vi "DIC main 11082010.vi"() -> ()   [LabVIEW 2010]
panel:
  in  "File Header Settings":T1={"Flow Rate"="", "Sample Volume"="", "Operator"="", "Sample Type"="Unknown"}
  in  "Sample Port":u16(ring) items=["A"=1, "B"=2, "C"=3, "D"=4, "E"=5, "F"=6, "G"=7, "H"=8]
  in  "flush syringe":bool
  in  "flush acid":bool
  in  "Syringe Flushes":i32=3
  out "file error out":errorcluster
  out "LiCor errors out":errorcluster
  out "kloehn errors out":errorcluster
  out "relay errors out":errorcluster
  out "Final Integral":dbl
  out "CO2 Integral":dbl
  out "pCO2_start":dbl
  out "pCO2_end":dbl
  in  "Start Run":bool caption="Make all inputs are set before hitting start!!!"
  in  "Number of Repeats":i32=1
  in  "stop":bool
  out "pCO2":dbl
  in  "Data Directory":path
  # "DIC Analysis Tool"
  # "Locate the directory where you would like to place your data files and then click \"Current Folder\""
  # "Global variables in Gernot's code:\nCO2pres\nCO2_Temp\nCom_Error\nCurrentRepeat\nDataFile\nError_Log\nH2O\nLicorData\nOperation\npCO2\npCO2_end\npCO2_integrate\npCO2_max\npCO2_start\nPeakAvg\nPeakRead\nRepeat\nSampleCount\nSampleID\nSampleTime\nSampleType\nSequenceTime\nSyringeCom\nTCO2Error\nValvePosition\nXplot\nYplot"
  # "Number of flushes before a sample is run or when Flush Syringe is pressed."
  # "Critical Points"
  # "Real Time"
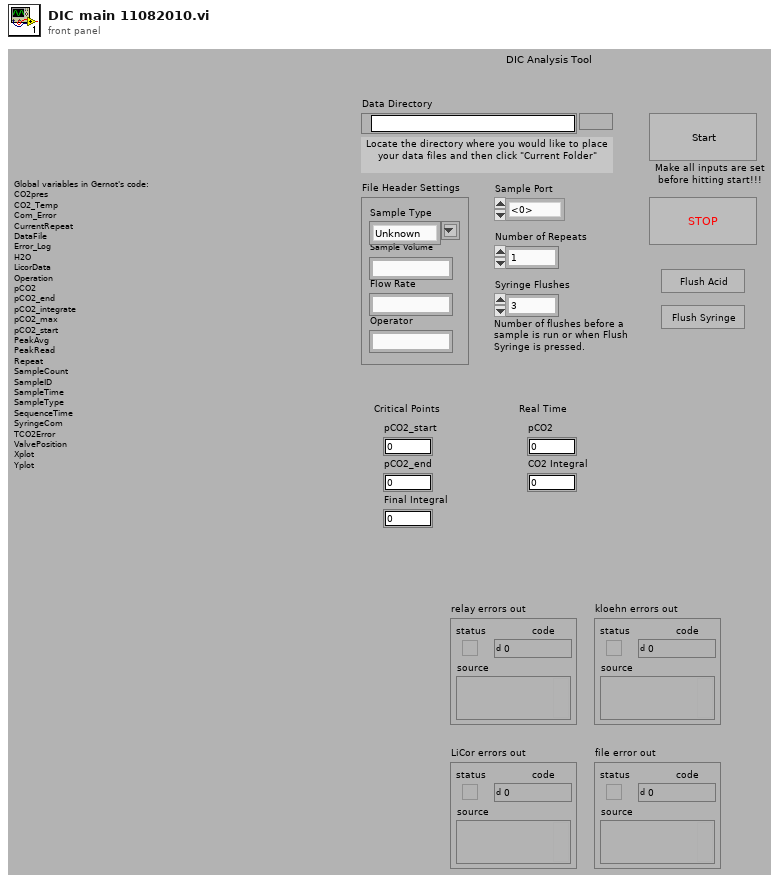
[diagram p1: front panel]
types:
  T1 = cluster{"Flow Rate":string, "Sample Volume":string, "Operator":string, "Sample Type":string}
  T2 = cluster{"baud rate (9600)":u32, "data bits (8)":u16, "parity (0:none)":enum16{"None", "Odd", "Even", "Mark", "Space"}, "stop bits (10: 1 bit)":u16, "flow control (0:none)":u16, "timeout (10sec)":u32, "termination char\n(0xA = '\\n' = LF) ":u8, "Enable Termination\nChar (T)":bool}
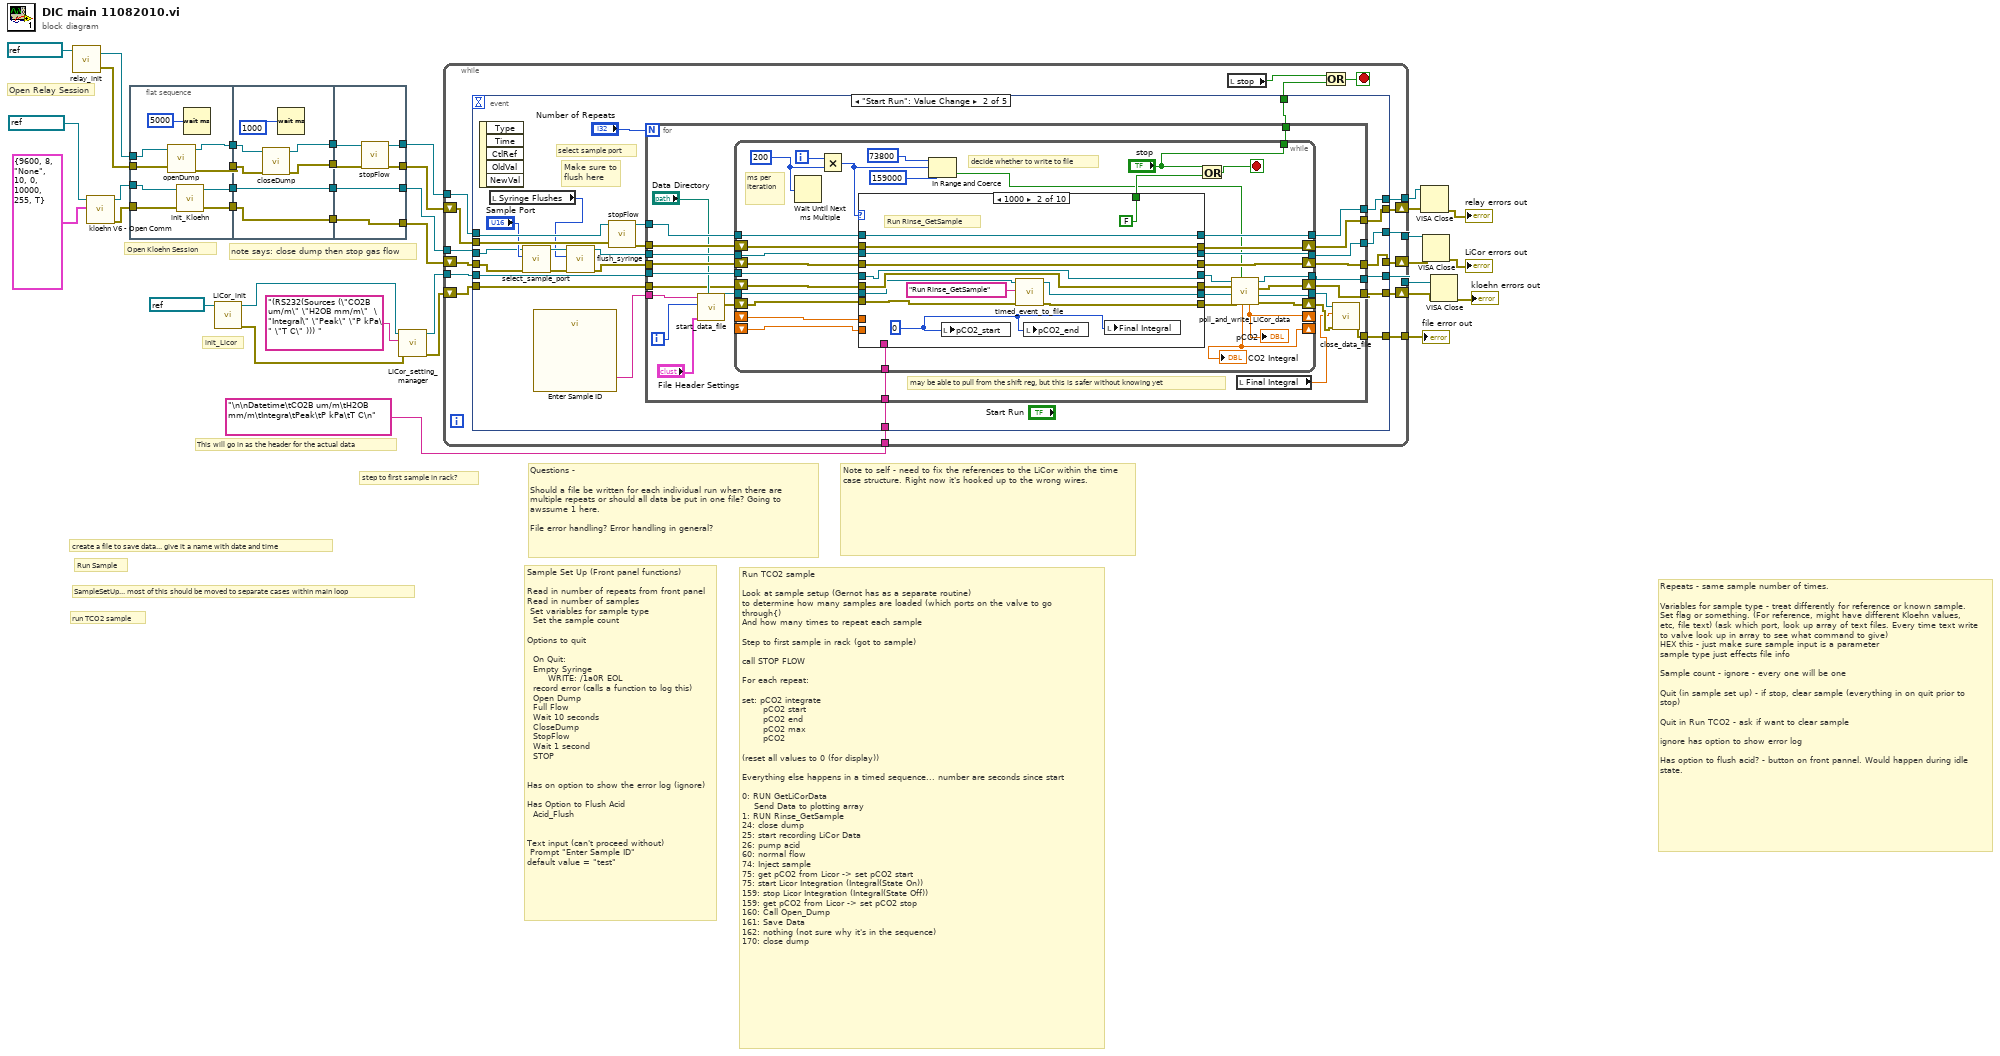
[diagram p0: block diagram]
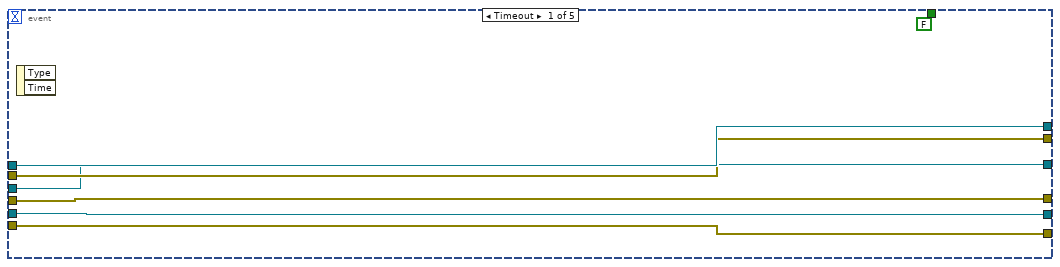
[diagram p2: hidden frame]
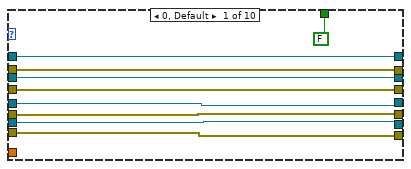
[diagram p3: hidden frame]
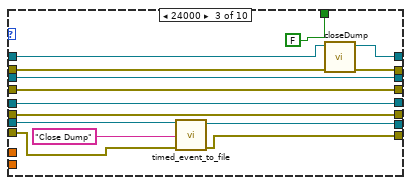
[diagram p4: hidden frame]
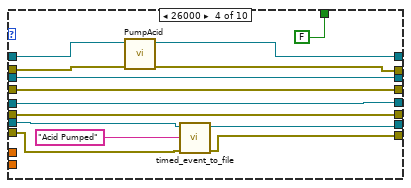
[diagram p5: hidden frame]
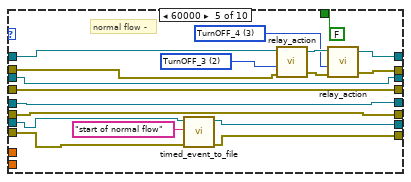
[diagram p6: hidden frame]
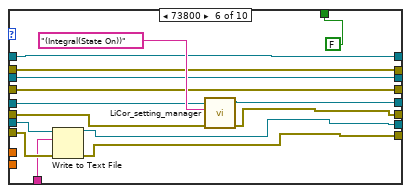
[diagram p7: hidden frame]
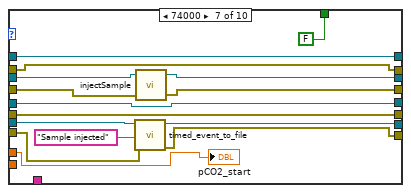
[diagram p8: hidden frame]
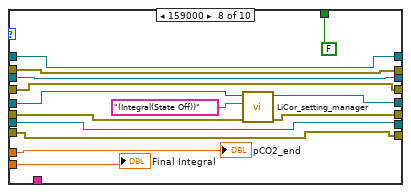
[diagram p9: hidden frame]
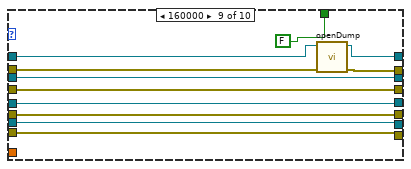
[diagram p10: hidden frame]
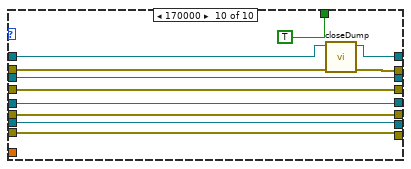
[diagram p11: hidden frame]
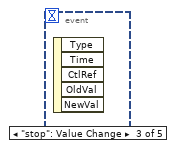
[diagram p12: hidden frame]
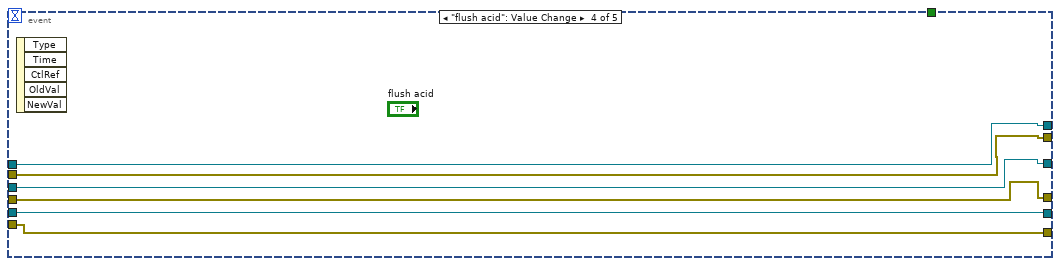
[diagram p13: hidden frame]
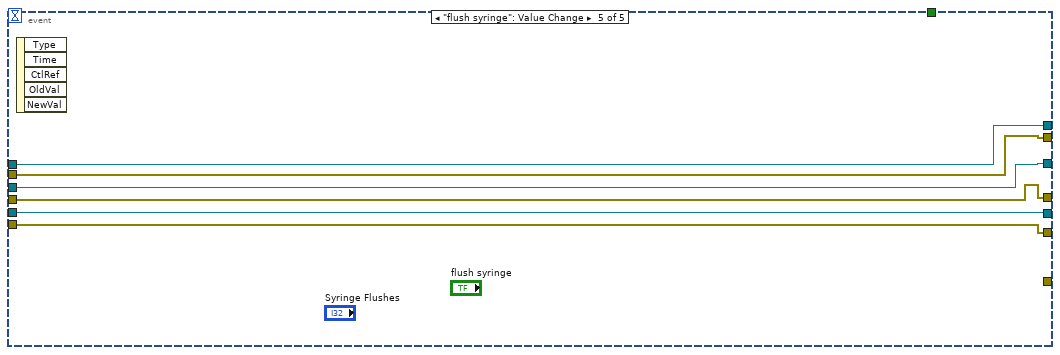
[diagram p14: hidden frame]
diagram:
  # "This will go in as the header for the actual data"
  # "step to first sample in rack?"
  # "Note to self - need to fix the references to the LiCor within the time case structure. Right now it's hooked up to the wrong wires."
  # "Questions - \n\nShould a file be written for each individual run when there are multiple repeats or should all data be put in one file? Going to awssume 1 here.\n\nFile error handling? Error handling in general?"
  # "Repeats - same sample number of times.\n\nVariables for sample type - treat differently for reference or known sample. Set flag or something. (For reference, might have different Kloehn values, etc, file text) (ask which port, look up array of text files. Every time text write to valve look up in array to see what command to give) \nHEX this - just make sure sample input is a parameter\nsample type just effects file info\n\nSample count - ignore - every one will be one\n\nQuit (in sample set up) - if stop, clear sample (everything in on quit prior to stop)\n\nQuit in Run TCO2 - ask if want to clear sample\n\nignore has option to show error log\n\nHas option to flush acid? - button on front pannel. Would happen during idle state."
  # "create a file to save data... give it a name with date and time"
  # "init_Licor"
  # "Run Sample"
  # "run TCO2 sample"
  # "SampleSetUp... most of this should be moved to separate cases within main loop"
  # "note says: close dump then stop gas flow"
  # "Open Relay Session"
  # "Open Kloehn Session"
  # "Run TCO2 sample\n\nLook at sample setup (Gernot has as a separate routine)\nto determine how many samples are loaded (which ports on the valve to go through{)\nAnd how many times to repeat each sample\n\nStep to first sample in rack (got to sample)\n\ncall STOP FLOW\n\nFor each repeat:\n\nset: pCO2 integrate\n       pCO2 start\n       pCO2 end\n       pCO2 max\n       pCO2 \n\n(reset all values to 0 (for display))\n\nEverything else happens in a timed sequence... number are seconds since start\n\n0: RUN GetLiCorData\n    Send Data to plotting array\n1: RUN Rinse_GetSample\n24: close dump\n25: start recording LiCor Data\n26: pump acid\n60: normal flow\n74: Inject sample\n75: get pCO2 from Licor -> set pCO2 start\n75: start Licor Integration (Integral(State On))\n159: stop Licor Integration (Integral(State Off))\n159: get pCO2 from Licor -> set pCO2 stop\n160: Call Open_Dump\n161: Save Data\n162: nothing (not sure why it's in the sequence)\n170: close dump"
  # "Sample Set Up (Front panel functions)\n\nRead in number of repeats from front panel\nRead in number of samples \n Set variables for sample type\n  Set the sample count\n\nOptions to quit\n\n  On Quit:\n  Empty Syringe \n       WRITE: /1a0R EOL\n  record error (calls a function to log this)\n  Open Dump\n  Full Flow\n  Wait 10 seconds\n  CloseDump\n  StopFlow\n  Wait 1 second\n  STOP\n\n\nHas on option to show the error log (ignore)\n\nHas Option to Flush Acid\n  Acid_Flush\n\n\nText input (can't proceed without)\n Prompt \"Enter Sample ID\"\ndefault value = \"test\""
  n1 = call "relay_init.vi"("VISA resource in"=refnum<visa-resource-name> "COM12" ("Koehn VISA Ref")) -> ("error out"=w35:errorcluster, "VISA resource out"=w36:refnum<visa-resource-name>)  [unwired: 2 in]
  n2 = call "kloehn V6 - Open Comm .vi"("Serial Parameters"=T2 {"baud rate (9600)"=9600, "data bits (8)"=8, "parity (0:none)"=enum."None", "stop bits (10: 1 bit)"=10, "flow control (0:none)"=0, "timeout (10sec)"=10000, "termination char\n(0xA = '\\n' = LF) "=255, "Enable Termination\nChar (T)"=TRUE} ("Port Configuration"), "VISA Ref in"=refnum<visa-resource-name> "COM10" ("Koehn VISA Ref")) -> ("error out"=w30:errorcluster, "VISA Ref out"=w31:refnum<visa-resource-name>)  [unwired: 8 in]
  n3 = flat-sequence {
    tunnel: w36 -> [w45]
    tunnel: w35 -> [w44]
    tunnel: [w43] -> w34
    tunnel: [w42] -> w33
    tunnel: w31 -> [w41]
    tunnel: w30 -> [w40]
    tunnel: [w39] -> w29
    tunnel: [w38] -> w28
    tunnel: w34 -> [w52]
    tunnel: w33 -> [w51]
    tunnel: w29 -> [w47]
    tunnel: w28 -> [w46]
    tunnel: [w50] -> w25
    tunnel: [w49] -> w24
    tunnel: [w47] -> w15
    tunnel: [w46] -> w14
    tunnel: w25 -> [w57]
    tunnel: w24 -> [w58]
    tunnel: [w56] -> w17
    tunnel: [w55] -> w16
    tunnel: w15 -> [w54]
    tunnel: w14 -> [w53]
    tunnel: [w54] -> w13
    tunnel: [w53] -> w12
    frame #0 {
      n4 = call "openDump.vi"("error in"=w44, "VISA resource name"=w45) -> ("error out"=w42:errorcluster, "VISA resource out"=w43:refnum<visa-resource-name>)  [unwired: 8 in]
      n5 = call "init_Kloehn.vi"("error in"=w40, "VISA resource in"=w41) -> ("error out"=w38:errorcluster, "VISA resource out"=w39:refnum<visa-resource-name>)  [unwired: 2 in]
      n6 = Wait (ms)(milliseconds to wait=5000) -> ()  [unwired: 1 out]
    }
    frame #1 {
      n7 = call "closeDump.vi"("error in"=w51, "VISA resource name"=w52) -> ("error out"=w50:errorcluster, "VISA resource out"=w49:refnum<visa-resource-name>)  [unwired: 8 in]
      n8 = Wait (ms)(milliseconds to wait=1000) -> ()  [unwired: 1 out]
    }
    frame #2 {
      n9 = call "stopFlow.vi"("error in"=w57, "VISA resource name"=w58) -> ("error out"=w55:errorcluster, "VISA resource out"=w56:refnum<visa-resource-name>)  [unwired: 8 in]
    }
  }
  n10 = call "LiCor_init.vi"("VISA resource name"=refnum<visa-resource-name> "COM11" ("Koehn VISA Ref")) -> ("error out"=w20:errorcluster, "VISA out"=w21:refnum<visa-resource-name>)  [unwired: 9 in]
  n11 = call "LiCor_setting_manager.vi"("error in"=w20, "string to write"="(RS232(Sources (\"CO2B um/m\" \"H2OB mm/m\"  \"Integral\" \"Peak\" \"P kPa\" \"T C\" ))) " ("String"), "VISA session in"=w21) -> ("error out"=w18:errorcluster, "VISA session out"=w19:refnum<visa-resource-name>)  [unwired: 7 in]
  n12 = while {
    tunnel: w19 -> [w63]
    tunnel: w17 -> [w75]
    tunnel: w13 -> [w73]
    tunnel: [w69] -> w10
    tunnel: [w68] -> w9
    tunnel: [w66] -> w7
    tunnel: "\n\nDatetime\tCO2B um/m\tH2OB mm/m\tIntegra\tPeak\tP kPa\tT C\n" -> [w60]
    tunnel: [w59] -> w4
    shift-right: [w70] -> w11
    shift-left: w18 -> [w64]
    shift-right: [w65] -> w6
    shift-left: w12 -> [w72]
    shift-right: [w67] -> w8
    shift-left: w16 -> [w74]
    stop <- w71 stop-if-true
    n13 = event shown="[1] \"Start Run\": Value Change" {
      selector: _ -> [_ _ _ _ _]
      dyn-events: _ -> [_ _ _ _ _]
      timeout: _ -> [_ _ _ _ _]
      tunnel: w63 -> [w81 w106 _ w301 w307]
      tunnel: w64 -> [w82 w105 _ w300 w306]
      tunnel: w75 -> [w80 w102 _ w305 w311]
      tunnel: w74 -> [w79 w101 _ w304 w310]
      tunnel: w73 -> [w78 w89 _ w303 w309]
      tunnel: w72 -> [w77 w88 _ w302 w308]
      tunnel: [FALSE w100 _ _ _] -> w61
      tunnel: [w82 w99 _ w300 w306] -> w70
      tunnel: [w81 w94 _ w301 w307] -> w69
      tunnel: [w80 w98 _ w305 w311] -> w68
      tunnel: [w79 w97 _ w304 w310] -> w67
      tunnel: [w78 w96 _ w303 w309] -> w66
      tunnel: [w77 w95 _ w302 w308] -> w65
      tunnel: w60 -> [_ w93 _ _ _]
      tunnel: [_ w91 _ _ _] -> w59
      event Timeout {
        n14 = event-data() -> ()  [unwired: 1 in, 2 out]
      }
      event "Start Run": Value Change {
        # "select sample port"
        # "Make sure to flush here"
        n15 = event-data() -> ()  [unwired: 1 in, 5 out]
        n16 = local read "Syringe Flushes"() -> (w83:i32)
        n17 = call "select_sample_port.vi"("error in"=w88, "Sample Port"="Sample Port", "VISA resource in"=w89) -> ("error out"=w87:errorcluster, "VISA resource out"=w86:refnum<visa-resource-name>)  [unwired: 7 in]
        n18 = call "Enter Sample ID"() -> ("sample id"=w92:string)  [unwired: 17 in, 2 out]
        n19 = call "flush_syringe.vi"("error in"=w87, "Syringe Flushes"=w83, "VISA resource in"=w86) -> ("error out"=w84:errorcluster, "VISA resource out"=w85:refnum<visa-resource-name>)  [unwired: 7 in]
        n20 = call "stopFlow.vi"("error in"=w101, "VISA resource name"=w102) -> ("error out"=w103:errorcluster, "VISA resource out"=w104:refnum<visa-resource-name>)  [unwired: 8 in]
        n21 = for {
          N: "Number of Repeats" -> [_]
          tunnel: w106 -> [w131]
          tunnel: w105 -> [w113]
          tunnel: w104 -> [w129]
          tunnel: w103 -> [w130]
          tunnel: [w128] -> w100
          tunnel: w85 -> [w127]
          tunnel: w84 -> [w126]
          tunnel: [w125] -> w99
          tunnel: [w124] -> w98
          tunnel: [w123] -> w97
          tunnel: [w122] -> w96
          tunnel: [w121] -> w95
          tunnel: [w120] -> w94
          tunnel: w92 -> [w116]
          tunnel: w93 -> [w117]
          tunnel: [w109] -> w91
          i -> [w114]
          # "may be able to pull from the shift reg, but this is safer without knowing yet"
          n22 = call "start_data_file.vi"("DataFile"="Data Directory", "File Header Settings"="File Header Settings", "iteration"=w114, "sample id"=w116) -> ("error out"=w118:errorcluster, "Byte Stream File Refnum"=w119:refnum<file>)  [unwired: 6 in]
          n23 = while {
            tunnel: w131 -> [w151]
            shift-right: [w140] -> w125
            shift-left: w113 -> [w150]
            tunnel: w129 -> [w165]
            shift-right: [w138] -> w111
            shift-left: w118 -> [w148]
            tunnel: ["stop"] -> w128
            tunnel: w127 -> [w163]
            shift-right: [w161] -> w121
            shift-left: w126 -> [w162]
            tunnel: [w160] -> w122
            tunnel: [w159] -> w124
            shift-right: [w158] -> w123
            shift-left: w130 -> [w164]
            tunnel: [w141] -> w120
            tunnel: w119 -> [w149]
            tunnel: [w139] -> w112
            tunnel: w117 -> [w152]
            shift-right: [w135] -> _
            shift-left: _ -> [w134]
            shift-right: [w133] -> _
            shift-left: _ -> [w132]
            i -> [w157]
            stop <- w153 stop-if-true
            w156 = 200 ("ms between samples")
            # "decide whether to write to file"
            # "ms per iteration"
            n24 = Wait Until Next ms Multiple(millisecond multiple=w156) -> ()  [unwired: 1 out]
            n25 = Multiply(x=w157, y=w156) -> (x*y=w136:i32)
            n26 = case shown="1000" w136 {
              tunnel: w165 -> [w166 w185 w199 w213 w225 w239 w263 w274 w286 w297]
              tunnel: w164 -> [w172 w184 w197 w212 w224 w240 w262 w273 w285 w296]
              tunnel: w163 -> [w174 w187 w200 w215 w233 w241 w261 w277 w288 w299]
              tunnel: w162 -> [w173 w186 w201 w214 w232 w242 w260 w276 w287 w298]
              tunnel: [w173 w186 w201 w214 w232 w242 w258 w276 w287 w298] -> w161
              tunnel: [w174 w187 w200 w215 w233 w241 w259 w277 w288 w299] -> w160
              tunnel: [w166 w185 w198 w211 w223 w239 w263 w274 w283 w294] -> w159
              tunnel: [w172 w184 w196 w210 w222 w240 w262 w273 w284 w295] -> w158
              tunnel: w151 -> [w170 w183 w195 w209 w231 w244 w256 w272 w282 w293]
              tunnel: w150 -> [w169 w182 w194 w208 w230 w243 w257 w271 w281 w292]
              tunnel: [w169 w182 w194 w208 w230 w236 w257 w269 w281 w292] -> w142
              tunnel: [w170 w183 w195 w209 w231 w237 w256 w270 w282 w293] -> w144
              tunnel: w149 -> [w168 w180 w191 w205 w219 w246 w253 w267 w279 w290]
              tunnel: [w167 w178 w188 w202 w217 w234 w250 w266 w278 w289] -> w143
              tunnel: w148 -> [w167 w179 w190 w204 w216 w248 w252 w266 w278 w289]
              tunnel: [w168 w177 w189 w203 w218 w235 w251 w267 w279 w290] -> w145
              tunnel: [FALSE FALSE FALSE FALSE FALSE FALSE FALSE FALSE FALSE TRUE] -> w155
              tunnel: w152 -> [_ _ _ _ _ w247 _ _ _ _]
              tunnel: w134 -> [_ _ _ _ _ _ w249 w265 _ _]
              tunnel: w132 -> [_ _ _ _ _ _ _ w264 _ _]
              frame 0, Default {
              }
              frame 1000 {
                w175 = 0
                # "Run Rinse_GetSample"
                n27 = local write "pCO2_start"(w175) -> ()
                n28 = call "timed_event_to_file.vi"("file error in"=w179, "String"="Run Rinse_GetSample", "file ref in"=w180) -> ("file error out"=w178:errorcluster, "file ref out"=w177:refnum<file>)  [unwired: 7 in]
                n29 = local write "pCO2_end"(w175) -> ()
                n30 = local write "Final Integral"(w175) -> ()
              }
              frame 24000 {
                n31 = call "timed_event_to_file.vi"("file error in"=w190, "String"="Close Dump", "file ref in"=w191) -> ("file error out"=w188:errorcluster, "file ref out"=w189:refnum<file>)  [unwired: 7 in]
                n32 = call "closeDump.vi"("error in"=w197, "VISA resource name"=w199) -> ("error out"=w196:errorcluster, "VISA resource out"=w198:refnum<visa-resource-name>)  [unwired: 8 in]
              }
              frame 26000 {
                n33 = call "PumpAcid.vi"("error in"=w212, "VISA resource name"=w213) -> ("error out"=w210:errorcluster, "VISA resource out"=w211:refnum<visa-resource-name>)  [unwired: 8 in]
                n34 = call "timed_event_to_file.vi"("file error in"=w204, "String"="Acid Pumped", "file ref in"=w205) -> ("file error out"=w202:errorcluster, "file ref out"=w203:refnum<file>)  [unwired: 7 in]
              }
              frame 60000 {
                w226 = u8 3 items=["TurnON_1"=8, "TurnON_PUMP"=9, "TurnON_3"=10, "TurnON_4"=11, "CLOSE DUMP OFF_1"=0, "TurnOFF_PUMP"=1, "TurnOFF_3"=2, "TurnOFF_4"=3, "OpenAll"=30, "CloseAllRelay"=29] ("Action 2")
                w229 = u8 2 items=["TurnON_1"=8, "TurnON_PUMP"=9, "TurnON_3"=10, "TurnON_4"=11, "CLOSE DUMP OFF_1"=0, "TurnOFF_PUMP"=1, "TurnOFF_3"=2, "TurnOFF_4"=3, "OpenAll"=30, "CloseAllRelay"=29] ("Action")
                # "normal flow -"
                n35 = call "timed_event_to_file.vi"("file error in"=w216, "String"="start of normal flow", "file ref in"=w219) -> ("file error out"=w217:errorcluster, "file ref out"=w218:refnum<file>)  [unwired: 7 in]
                n36 = call "relay_action.vi"("VISA resource in"=w225, "Action"=w229, "error in"=w224) -> ("VISA resource out"=w228:refnum<visa-resource-name>, "error out"=w227:errorcluster)  [unwired: 4 in]
                n37 = call "relay_action.vi"("VISA resource in"=w228, "Action"=w226, "error in"=w227) -> ("VISA resource out"=w223:refnum<visa-resource-name>, "error out"=w222:errorcluster)  [unwired: 4 in]
              }
              frame 73800 {
                n38 = Write to Text File(file (use dialog)=w246, text=w247, error in=w248) -> (refnum out=w235:refnum<file>, error out=w234:errorcluster)  [unwired: 1 in, 1 out]
                n39 = call "LiCor_setting_manager.vi"("error in"=w243, "string to write"="(Integral(State On))", "VISA session in"=w244) -> ("error out"=w236:errorcluster, "VISA session out"=w237:refnum<visa-resource-name>)  [unwired: 7 in]
              }
              frame 74000 {
                n40 = call "timed_event_to_file.vi"("file error in"=w252, "String"="Sample injected", "file ref in"=w253) -> ("file error out"=w250:errorcluster, "file ref out"=w251:refnum<file>)  [unwired: 7 in]
                n41 = call "injectSample.vi"("error in"=w260, "VISA resource in"=w261) -> ("error out"=w258:errorcluster, "VISA resource out"=w259:refnum<visa-resource-name>)  [unwired: 2 in]
                "pCO2_start" <- w249
              }
              frame 159000 {
                n42 = call "LiCor_setting_manager.vi"("error in"=w271, "string to write"="(Integral(State Off))", "VISA session in"=w272) -> ("error out"=w269:errorcluster, "VISA session out"=w270:refnum<visa-resource-name>)  [unwired: 7 in]
                "pCO2_end" <- w265
                "Final Integral" <- w264
              }
              frame 160000 {
                n43 = call "openDump.vi"("error in"=w285, "VISA resource name"=w286) -> ("error out"=w284:errorcluster, "VISA resource out"=w283:refnum<visa-resource-name>)  [unwired: 8 in]
              }
              frame 170000 {
                n44 = call "closeDump.vi"("error in"=w296, "VISA resource name"=w297) -> ("error out"=w295:errorcluster, "VISA resource out"=w294:refnum<visa-resource-name>)  [unwired: 8 in]
              }
            }
            n45 = In Range and Coerce(upper limit=73800, x=w136, lower limit=159000) -> (In Range?=w137:bool)  [unwired: 1 out]
            n46 = Or(x="stop", y=w155) -> (x .or. y?=w153:bool)
            n47 = call "poll_and_write_LiCor_data.vi"("write to file?"=w137, "file error in"=w143, "file ref in"=w145, "LiCor error in"=w142, "LiCor session in"=w144) -> ("file error out"=w138:errorcluster, "file ref out"=w139:refnum<file>, "LiCor error out"=w140:errorcluster, "LiCor session out"=w141:refnum<visa-resource-name>, "pCO2"=w135:dbl, "CO2 integral"=w133:dbl)  [unwired: 1 in]
            "pCO2" <- w135
            "CO2 Integral" <- w133
          }
          n48 = local read "Final Integral"() -> (w110:dbl)
          n49 = call "close_data_file.vi"("error in"=w111, "Final integral"=w110, "file refnum in"=w112) -> ("error out"=w109:errorcluster)  [unwired: 7 in, 1 out]
        }
      }
      event "stop": Value Change {
        n50 = event-data() -> ()  [unwired: 1 in, 5 out]
      }
      event "flush acid": Value Change {
        n51 = event-data() -> ()  [unwired: 1 in, 5 out]
      }
      event "flush syringe": Value Change {
        n52 = event-data() -> ()  [unwired: 1 in, 5 out]
      }
    }
    n53 = local read "stop"() -> (w62:bool)
    n54 = Or(x=w62, y=w61) -> (x .or. y?=w71:bool)
  }
  "file error out" <- w4
  n55 = VISA Close(VISA resource name=w9, error in (no error)=w8) -> (error out=→"relay errors out":errorcluster)
  n56 = VISA Close(VISA resource name=w7, error in (no error)=w6) -> (error out=→"LiCor errors out":errorcluster)
  n57 = VISA Close(VISA resource name=w10, error in (no error)=w11) -> (error out=→"kloehn errors out":errorcluster)
